vi "Play Alarm.vi"(8 "error in (no error)":errorcluster, 11 "Controller in":refnum<class "Controller.lvclass">) -> (0 "error out":errorcluster, 3 "Controller out":refnum<class "Controller.lvclass">)   [LabVIEW 2016, in "Controller Actor.lvlib" / "Controller.lvclass"]
uses:
  <userlib>/Common Components/Controller/Controller.lvclass
  <userlib>/Common Components/Common/Common.lvlib
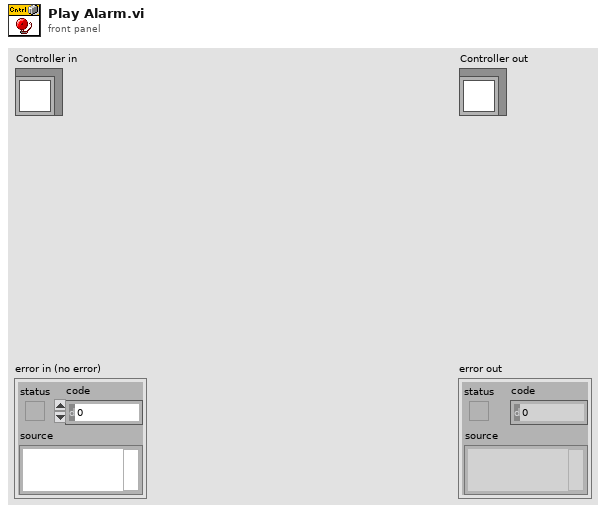
[diagram p1: front panel]
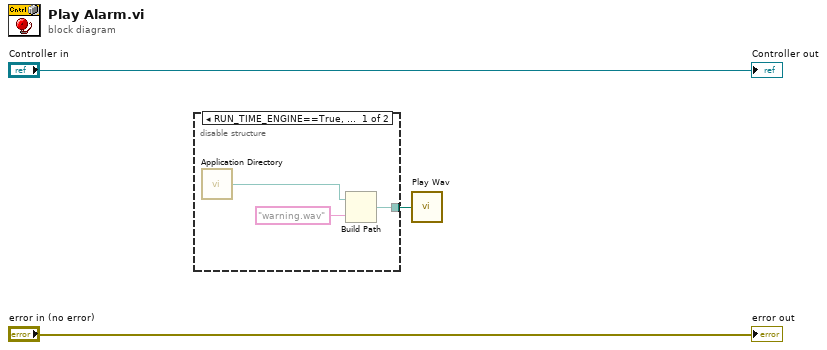
[diagram p0: block diagram]
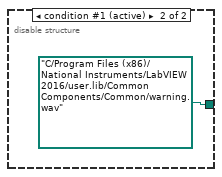
[diagram p2: hidden frame]
diagram:
  n1 = disable-structure shown="RUN_TIME_ENGINE==True, Default" {
    disable-tunnel: [w4 path "C:/Program Files (x86)/National Instruments/LabVIEW 2016/user.lib/Common Components/Common/warning.wav" ("Path")] -> w1
    frame condition #0 {
      n2 = call <vilib>:"Application Directory.vi"() -> ("Application Directory"=w6:path)
      n3 = Build Path(base path=w6, name or relative path="warning.wav") -> (appended path=w4:path)
    }
    frame condition #1 (active) {
    }
  }
  n4 = call <userlib>:"Play Wav.vi"("path"=w1) -> ()  [unwired: 1 out]
  "error out" <- "error in (no error)"
  "Controller out" <- "Controller in"
